vi "rsidr_core_global.vi"() -> ()   [LabVIEW 2020, in "Rohde&Schwarz RTx Oscilloscopes.lvlib"] (continued)
"Data Type"=0, "Command"="", "Access"=0, "Range Table"="", "Read Callback"="", "Write Callback"="", "Supported Models"="", "Instrument Options"="", "Flags"=0, "Help"="Current harmonics measurement total harmonic distortion results."}, {"Level"=4, "Class Only"=FALSE, "Identifier"="RSRTX_ATTR_POWER_CURRENT_HARMONICS_MEASUREMENT_TOTAL_HARMONIC_DISTORTION_CURRENT", "Descriptive Name"="Power Current Harmonics Measurement Total Harmonic Distortion Current", "Data Type"=1, "Command"="POW:HARM:MEAS:THD?", "Access"=0, "Range Table"="", "Read Callback"="", "Write Callback"="", "Supported Models"="RTM|RTA", "Instrument Options"="", "Flags"=0, "Help"="Returns the current total harmonic disortion value.\n\nAvailable Repeated Capabilities:\nNone\n\nRemote-control command(s):\nPOWer:HARMonics:MEASurement:THDistortion[:ACTual]?"}, {"Level"=4, "Class Only"=FALSE, "Identifier"="RSRTX_ATTR_POWER_CURRENT_HARMONICS_MEASUREMENT_TOTAL_HARMONIC_DISTORTION_AVERAGE", "Descriptive Name"="Power Current Harmonics Measurement Total Harmonic Distortion Average", "Data Type"=1, "Command"="POW:HARM:MEAS:THD:AVG?", "Access"=0, "Range Table"="", "Read Callback"="", "Write Callback"="", "Supported Models"="RTM|RTA", "Instrument Options"="", "Flags"=0, "Help"="Returns the average total harmonic disortion of the measured signal.\n\nAvailable Repeated Capabilities:\nNone\n\nRemote-control command(s):\nPOWer:HARMonics:MEASurement:THDistortion:AVG?"}, {"Level"=4, "Class Only"=FALSE, "Identifier"="RSRTX_ATTR_POWER_CURRENT_HARMONICS_MEASUREMENT_TOTAL_HARMONIC_DISTORTION_MAXIMUM", "Descriptive Name"="Power Current Harmonics Measurement Total Harmonic Distortion Maximum", "Data Type"=1, "Command"="POW:HARM:MEAS:THD:PPE?", "Access"=0, "Range Table"="", "Read Callback"="", "Write Callback"="", "Supported Models"="RTM|RTA", "Instrument Options"="", "Flags"=0, "Help"="Returns the maximum total harmonic disortion of the measured signal.\n\nAvailable Repeated Capabilities:\nNone\n\nRemote-control command(s):\nPOWer:HARMonics:MEASurement:THDistortion:PPEak?"}, {"Level"=4, "Class Only"=FALSE, "Identifier"="RSRTX_ATTR_POWER_CURRENT_HARMONICS_MEASUREMENT_TOTAL_HARMONIC_DISTORTION_MINIMUM", "Descriptive Name"="Power Current Harmonics Measurement Total Harmonic Distortion Minimum", "Data Type"=1, "Command"="POW:HARM:MEAS:THD:NPE?", "Access"=0, "Range Table"="", "Read Callback"="", "Write Callback"="", "Supported Models"="RTM|RTA", "Instrument Options"="", "Flags"=0, "Help"="Returns the minimum total harmonic disortion of the measured signal.\n\nAvailable Repeated Capabilities:\nNone\n\nRemote-control command(s):\nPOWer:HARMonics:MEASurement:THDistortion:NPEak?"}, {"Level"=4, "Class Only"=FALSE, "Identifier"="RSRTX_ATTR_POWER_CURRENT_HARMONICS_MEASUREMENT_TOTAL_HARMONIC_DISTORTION_STANDARD_DEVIATION", "Descriptive Name"="Power Current Harmonics Measurement Total Harmonic Distortion Standard Deviation", "Data Type"=1, "Command"="POW:HARM:MEAS:THD:STDD?", "Access"=0, "Range Table"="", "Read Callback"="", "Write Callback"="", "Supported Models"="RTM|RTA", "Instrument Options"="", "Flags"=0, "Help"="Returns the standard deviation of total harmonic disortions of the measured signal.\n\nAvailable Repeated Capabilities:\nNone\n\nRemote-control command(s):\nPOWer:HARMonics:MEASurement:THDistortion:STDDev?"}, {"Level"=3, "Class Only"=TRUE, "Identifier"="", "Descriptive Name"="Current Harmonics Export", "Data Type"=0, "Command"="", "Access"=0, "Range Table"="", "Read Callback"="", "Write Callback"="", "Supported Models"="", "Instrument Options"="", "Flags"=0, "Help"="Contains attributes for eporting power measurement."}, {"Level"=4, "Class Only"=FALSE, "Identifier"="RSRTX_ATTR_CURRENT_HARMONICS_EXPORT_NAME", "Descriptive Name"="Current Harmonics Export Name", "Data Type"=2, "Command"="EXP:POW:NAME", "Access"=2, "Range Table"="", "Read Callback"="", "Write Callback"="", "Supported Models"="RTM|RTA", "Instrument Options"="", "Flags"=0, "Help"="Defines the path and filename of the results file, available for current harmonics and spectrum power measurements. The file format is CSV. If the file already exists, it will be overwritten.\n\nAvailable Repeated Capabilities:\nNone\n\nRemote-control command(s):\nEXPort:POWer:NAME"}, {"Level"=4, "Class Only"=FALSE, "Identifier"="RSRTX_ATTR_CURRENT_HARMONICS_EXPORT_SAVE", "Descriptive Name"="Current Harmonics Export Save", "Data Type"=4, "Command"="EXP:POW:SAVE", "Access"=1, "Range Table"="", "Read Callback"="", "Write Callback"="", "Supported Models"="RTM|RTA", "Instrument Options"="", "Flags"=0, "Help"="Saves statistical results of the indicated measurement place to the file that is defined by RSRTX_ATTR_CURRENT_HARMONICS_EXPORT_NAME.\n\nAvailable Repeated Capabilities:\nNone\n\nRemote-control command(s):\nEXPort:POWer:SAVE"}, {"Level"=2, "Class Only"=TRUE, "Identifier"="", "Descriptive Name"="Inrush Current Measurement", "Data Type"=0, "Command"="", "Access"=0, "Range Table"="", "Read Callback"="", "Write Callback"="", "Supported Models"="", "Instrument Options"="", "Flags"=0, "Help"="Inrush current measurement."}, {"Level"=3, "Class Only"=FALSE, "Identifier"="RSRTX_ATTR_START_POWER_INRUSH_CURRENT_MEASUREMENT", "Descriptive Name"="Start Power Inrush Current Measurement", "Data Type"=4, "Command"="POW:INR:EXEC", "Access"=1, "Range Table"="", "Read Callback"="", "Write Callback"="", "Supported Models"="RTM|RTA", "Instrument Options"="", "Flags"=0, "Help"="Start power inrush current measurement.\n\nAvailable Repeated Capabilities:\nNone\n\nRemote-control command(s):\nPOWer:INRushcurrent:EXECute"}, {"Level"=3, "Class Only"=FALSE, "Identifier"="RSRTX_ATTR_POWER_INRUSH_CURRENT_MEASUREMENT_GATE_COUNT", "Descriptive Name"="Power Inrush Current Measurement Gate Count", "Data Type"=0, "Command"="POW:INR:GCO", "Access"=2, "Range Table"="", "Read Callback"="", "Write Callback"="", "Supported Models"="RTM|RTA", "Instrument Options"="", "Flags"=0, "Help"="Power inrush current measurement gate count.\n\nAvailable Repeated Capabilities:\nNone\n\nRemote-control command(s):\nPOWer:INRushcurrent:GCOunt"}, {"Level"=3, "Class Only"=FALSE, "Identifier"="RSRTX_ATTR_POWER_INRUSH_CURRENT_MEASUREMENT_ADD_REPORT", "Descriptive Name"="Power Inrush Current Measurement Add Report", "Data Type"=4, "Command"="POW:INR:REP:ADD", "Access"=1, "Range Table"="", "Read Callback"="", "Write Callback"="", "Supported Models"="RTM|RTA", "Instrument Options"="", "Flags"=1, "Help"="Adds the result to the report list.\n\nAvailable Repeated Capabilities:\nNone\n\nRemote-control command(s):\nPOWer:INRushcurrent:REPort:ADD"}, {"Level"=3, "Class Only"=TRUE, "Identifier"="", "Descriptive Name"="Gate", "Data Type"=0, "Command"="", "Access"=0, "Range Table"="", "Read Callback"="", "Write Callback"="", "Supported Models"="", "Instrument Options"="", "Flags"=0, "Help"="Attributes with gate repeated capability."}, {"Level"=4, "Class Only"=FALSE, "Identifier"="RSRTX_ATTR_POWER_INRUSH_CURRENT_MEASUREMENT_GATE_START", "Descriptive Name"="Power Inrush Current Measurement Gate Start", "Data Type"=1, "Command"="POW:INR:GATE{Gate}:STAR", "Access"=2, "Range Table"="", "Read Callback"="", "Write Callback"="", "Supported Models"="RTM|RTA", "Instrument Options"="", "Flags"=0, "Help"="Start of the gate.\n\nAvailable Repeated Capabilities:\nGate: Gate1, Gate2, Gate3\r\n\nRemote-control command(s):\nPOWer:INRushcurrent:GATE<n>:STARt"}, {"Level"=4, "Class Only"=FALSE, "Identifier"="RSRTX_ATTR_POWER_INRUSH_CURRENT_MEASUREMENT_GATE_STOP", "Descriptive Name"="Power Inrush Current Measurement Gate Stop", "Data Type"=1, "Command"="POW:INR:GATE{Gate}:STOP", "Access"=2, "Range Table"="", "Read Callback"="", "Write Callback"="", "Supported Models"="RTM|RTA", "Instrument Options"="", "Flags"=0, "Help"="Stop of the gate.\n\nAvailable Repeated Capabilities:\nGate: Gate1, Gate2, Gate3\r\n\nRemote-control command(s):\nPOWer:INRushcurrent:GATE<n>:STOP"}, {"Level"=3, "Class Only"=TRUE, "Identifier"="", "Descriptive Name"="Results", "Data Type"=0, "Command"="", "Access"=0, "Range Table"="", "Read Callback"="", "Write Callback"="", "Supported Models"="", "Instrument Options"="", "Flags"=0, "Help"="Results of the inrush current measurement."}, {"Level"=4, "Class Only"=FALSE, "Identifier"="RSRTX_ATTR_POWER_INRUSH_CURRENT_MEASUREMENT_AREA_RESULT", "Descriptive Name"="Power Inrush Current Measurement Area Result", "Data Type"=1, "Command"="POW:INR:RES{Gate}:AREA?", "Access"=0, "Range Table"="", "Read Callback"="", "Write Callback"="", "Supported Models"="RTM|RTA", "Instrument Options"="", "Flags"=0, "Help"="Area result of the measurement.\n\nAvailable Repeated Capabilities:\nGate: Gate1, Gate2, Gate3\r\n\nRemote-control command(s):\nPOWer:INRushcurrent:RESult<n>:AREA?"}, {"Level"=4, "Class Only"=FALSE, "Identifier"="RSRTX_ATTR_POWER_INRUSH_CURRENT_MEASUREMENT_MAXIMUM_RESULT", "Descriptive Name"="Power Inrush Current Measurement Maximum Result", "Data Type"=1, "Command"="POW:INR:RES{Gate}:MAXCurrent?", "Access"=0, "Range Table"="", "Read Callback"="", "Write Callback"="", "Supported Models"="RTM|RTA", "Instrument Options"="", "Flags"=0, "Help"="Maximum result of the measurement.\n\nAvailable Repeated Capabilities:\nGate: Gate1, Gate2, Gate3\r\n\nRemote-control command(s):\nPOWer:INRushcurrent:RESult<n>:MAXCurrent?"}, {"Level"=2, "Class Only"=TRUE, "Identifier"="", "Descriptive Name"="Ripple Measurement", "Data Type"=0, "Command"="", "Access"=0, "Range Table"="", "Read Callback"="", "Write Callback"="", "Supported Models"="", "Instrument Options"="", "Flags"=0, "Help"="Ripple mesurement."}, {"Level"=3, "Class Only"=FALSE, "Identifier"="RSRTX_ATTR_START_POWER_RIPPLE_MEASUREMENT", "Descriptive Name"="Start Power Ripple Measurement", "Data Type"=4, "Command"="POW:RIPP:EXEC", "Access"=1, "Range Table"="", "Read Callback"="", "Write Callback"="", "Supported Models"="RTM|RTA", "Instrument Options"="", "Flags"=0, "Help"="Start power ripple measurement.\n\nAvailable Repeated Capabilities:\nNone\n\nRemote-control command(s):\nPOWer:RIPPle:EXECute"}, {"Level"=3, "Class Only"=FALSE, "Identifier"="RSRTX_ATTR_POWER_RIPPLE_MEASUREMENT_ADD_REPORT", "Descriptive Name"="Power Ripple Measurement Add Report", "Data Type"=4, "Command"="POW:RIPP:REP:ADD", "Access"=1, "Range Table"="", "Read Callback"="", "Write Callback"="", "Supported Models"="RTM|RTA", "Instrument Options"="", "Flags"=1, "Help"="Adds the result to the report list.\n\nAvailable Repeated Capabilities:\nNone\n\nRemote-control command(s):\nPOWer:RIPPle:REPort:ADD"}, {"Level"=3, "Class Only"=TRUE, "Identifier"="", "Descriptive Name"="Results", "Data Type"=0, "Command"="", "Access"=0, "Range Table"="", "Read Callback"="", "Write Callback"="", "Supported Models"="", "Instrument Options"="", "Flags"=0, "Help"="Results of the ripple analysis."}, {"Level"=2, "Class Only"=TRUE, "Identifier"="", "Descriptive Name"="Spectrum Measurement", "Data Type"=0, "Command"="", "Access"=0, "Range Table"="", "Read Callback"="", "Write Callback"="", "Supported Models"="", "Instrument Options"="", "Flags"=0, "Help"="Power spectrum measurement."}, {"Level"=3, "Class Only"=FALSE, "Identifier"="RSRTX_ATTR_START_POWER_SPECTRUM_MEASUREMENT", "Descriptive Name"="Start Power Spectrum Measurement", "Data Type"=4, "Command"="POW:SPEC:EXEC", "Access"=1, "Range Table"="", "Read Callback"="", "Write Callback"="", "Supported Models"="RTM|RTA", "Instrument Options"="", "Flags"=1, "Help"="Starts the spectrum measurement.\n\nAvailable Repeated Capabilities:\nNone\n\nRemote-control command(s):\nPOWer:SPECtrum:EXECute"}, {"Level"=3, "Class Only"=FALSE, "Identifier"="RSRTX_ATTR_POWER_SPECTRUM_MEASUREMENT_FREQUENCY", "Descriptive Name"="Power Spectrum Measurement Frequency", "Data Type"=1, "Command"="POW:SPEC:FREQ", "Access"=2, "Range Table"="", "Read Callback"="", "Write Callback"="", "Supported Models"="RTM|RTA", "Instrument Options"="", "Flags"=0, "Help"="Sets the SMPS switching frequency.\n\nAvailable Repeated Capabilities:\nNone\n\nRemote-control command(s):\nPOWer:SPECtrum:FREQuency"}, {"Level"=3, "Class Only"=FALSE, "Identifier"="RSRTX_ATTR_POWER_SPECTRUM_MEASUREMENT_ADD_REPORT", "Descriptive Name"="Power Spectrum Measurement Add Report", "Data Type"=4, "Command"="POW:SPEC:REP:ADD", "Access"=1, "Range Table"="", "Read Callback"="", "Write Callback"="", "Supported Models"="RTM|RTA", "Instrument Options"="", "Flags"=1, "Help"="Adds the result to the report list.\n\nAvailable Repeated Capabilities:\nNone\n\nRemote-control command(s):\nPOWer:SPECtrum:REPort:ADD"}, {"Level"=3, "Class Only"=TRUE, "Identifier"="", "Descriptive Name"="Results", "Data Type"=0, "Command"="", "Access"=0, "Range Table"="", "Read Callback"="", "Write Callback"="", "Supported Models"="", "Instrument Options"="", "Flags"=0, "Help"="Power Spectrum Measurement Results."}, {"Level"=4, "Class Only"=FALSE, "Identifier"="RSRTX_ATTR_RESET_POWER_SPECTRUM_MEASUREMENT_RESULTS", "Descriptive Name"="Reset Power Spectrum Measurement Results", "Data Type"=4, "Command"="POW:SPEC:RES{ResultNumber}:RES", "Access"=1, "Range Table"="", "Read Callback"="", "Write Callback"="", "Supported Models"="RTM|RTA", "Instrument Options"="", "Flags"=0, "Help"="Resets the results.\n\nAvailable Repeated Capabilities:\nResultNumber: Res1, Res2, Res3, Res4, Res5, Res6, Res7, Res8, Res9, Res10, Res11, Res12, Res13, Res14, Res15, Res16, Res17, Res18, Res19, Res20, Res21, Res22, Res23, Res24, Res25, Res26, Res27, Res28, Res29, Res30, Res31, Res32, Res33, Res34, Res35, Res36, Res37, Res38, Res39, Res40\r\n\nRemote-control command(s):\nPOWer:SPECtrum:RESult<n>:RESet"}, {"Level"=2, "Class Only"=TRUE, "Identifier"="", "Descriptive Name"="Slew Rate Measurement", "Data Type"=0, "Command"="", "Access"=0, "Range Table"="", "Read Callback"="", "Write Callback"="", "Supported Models"="", "Instrument Options"="", "Flags"=0, "Help"="Slew rate measurement."}, {"Level"=3, "Class Only"=FALSE, "Identifier"="RSRTX_ATTR_START_POWER_SLEW_RATE_MEASUREMENT", "Descriptive Name"="Start Power Slew Rate Measurement", "Data Type"=4, "Command"="POW:SLEW:EXEC", "Access"=1, "Range Table"="", "Read Callback"="", "Write Callback"="", "Supported Models"="RTM|RTA", "Instrument Options"="", "Flags"=0, "Help"="Starts the slew rate measurement.\n\nAvailable Repeated Capabilities:\nNone\n\nRemote-control command(s):\nPOWer:SLEWrate:EXECute"}, {"Level"=3, "Class Only"=FALSE, "Identifier"="RSRTX_ATTR_POWER_SLEW_RATE_MEASUREMENT_DELTA_SAMPLE", "Descriptive Name"="Power Slew Rate Measurement Delta Sample", "Data Type"=1, "Command"="POW:SLEW:DSAM", "Access"=2, "Range Table"="", "Read Callback"="", "Write Callback"="", "Supported Models"="RTM|RTA", "Instrument Options"="", "Flags"=0, "Help"="Configures the length of the delta sample\n\nAvailable Repeated Capabilities:\nNone\n\nRemote-control command(s):\nPOWer:SLEWrate:DSAMple"}, {"Level"=3, "Class Only"=FALSE, "Identifier"="RSRTX_ATTR_POWER_SLEW_RATE_MEASUREMENT_DELTA_TIME", "Descriptive Name"="Power Slew Rate Measurement Delta Time", "Data Type"=1, "Command"="POW:SLEW:DTIM", "Access"=2, "Range Table"="", "Read Callback"="", "Write Callback"="", "Supported Models"="RTM|RTA", "Instrument Options"="", "Flags"=0, "Help"="Configures the delta time.\n\nAvailable Repeated Capabilities:\nNone\n\nRemote-control command(s):\nPOWer:SLEWrate:DTIMe"}, {"Level"=3, "Class Only"=FALSE, "Identifier"="RSRTX_ATTR_POWER_SLEW_RATE_MEASUREMENT_ADD_REPORT", "Descriptive Name"="Power Slew Rate Measurement Add Report", "Data Type"=4, "Command"="POW:SLEW:REP:ADD", "Access"=1, "Range Table"="", "Read Callback"="", "Write Callback"="", "Supported Models"="RTM|RTA", "Instrument Options"="", "Flags"=1, "Help"="Adds the result to the report list.\n\nAvailable Repeated Capabilities:\nNone\n\nRemote-control command(s):\nPOWer:SLEWrate:REPort:ADD"}, {"Level"=3, "Class Only"=TRUE, "Identifier"="", "Descriptive Name"="Results", "Data Type"=0, "Command"="", "Access"=0, "Range Table"="", "Read Callback"="", "Write Callback"="", "Supported Models"="", "Instrument Options"="", "Flags"=0, "Help"="Slew rate measurement results."}, {"Level"=2, "Class Only"=TRUE, "Identifier"="", "Descriptive Name"="Modulation Measurement", "Data Type"=0, "Command"="", "Access"=0, "Range Table"="", "Read Callback"="", "Write Callback"="", "Supported Models"="", "Instrument Options"="", "Flags"=0, "Help"="Power modulation measurement."}, {"Level"=3, "Class Only"=FALSE, "Identifier"="RSRTX_ATTR_START_POWER_MODULATION_MEASUREMENT", "Descriptive Name"="Start Power Modulation Measurement", "Data Type"=4, "Command"="POW:MOD:EXEC", "Access"=1, "Range Table"="", "Read Callback"="", "Write Callback"="", "Supported Models"="RTM|RTA", "Instrument Options"="", "Flags"=0, "Help"="Starts the measurement.\n\nAvailable Repeated Capabilities:\nNone\n\nRemote-control command(s):\nPOWer:MODulation:EXECute"}, {"Level"=3, "Class Only"=FALSE, "Identifier"="RSRTX_ATTR_POWER_MODULATION_MEASUREMENT_TYPE", "Descriptive Name"="Power Modulation Measurement Type", "Data Type"=0, "Command"="POW:MOD:TYPE", "Access"=2, "Range Table"="rsrtx_rngModulationType", "Read Callback"="", "Write Callback"="", "Supported Models"="RTM|RTA", "Instrument Options"="", "Flags"=0, "Help"="Selects modulation type.\n\nAvailable Repeated Capabilities:\nNone\n\nRemote-control command(s):\nPOWer:MODulation:TYPE"}, {"Level"=3, "Class Only"=FALSE, "Identifier"="RSRTX_ATTR_POWER_MODULATION_MEASUREMENT_ADD_REPORT", "Descriptive Name"="Power Modulation Measurement Add Report", "Data Type"=4, "Command"="POW:MOD:REP:ADD", "Access"=1, "Range Table"="", "Read Callback"="", "Write Callback"="", "Supported Models"="RTM|RTA", "Instrument Options"="", "Flags"=1, "Help"="Adds the result to the report list.\n\nAvailable Repeated Capabilities:\nNone\n\nRemote-control command(s):\nPOWer:MODulation:REPort:ADD"}, {"Level"=3, "Class Only"=FALSE, "Identifier"="RSRTX_ATTR_POWER_MODULATION_THRESHOLD_UPPER", "Descriptive Name"="Power Modulation Threshold Upper", "Data Type"=1, "Command"="POW:MOD:THR", "Access"=2, "Range Table"="", "Read Callback"="", "Write Callback"="", "Supported Models"="", "Instrument Options"="", "Flags"=0, "Help"="Sets the threshold for unipolar sources, or the upper level for bipolar sources. The signal is measured at the crossing points of the signal with the threshold.\n\nAvailable Repeated Capabilities:\nNone\n\nRemote-control command(s):\nPOWer:MODulation:THReshold[:UPPer]"}, {"Level"=3, "Class Only"=FALSE, "Identifier"="RSRTX_ATTR_POWER_MODULATION_THRESHOLD_LOWER", "Descriptive Name"="Power Modulation Threshold Lower", "Data Type"=1, "Command"="POW:MOD:THR:LOW", "Access"=2, "Range Table"="", "Read Callback"="", "Write Callback"="", "Supported Models"="", "Instrument Options"="", "Flags"=0, "Help"="Sets the lower level for bipolar sources, which determines the crossing points on negative pulses.\n\nAvailable Repeated Capabilities:\nNone\n\nRemote-control command(s):\nPOWer:MODulation:THReshold:LOWer"}, {"Level"=3, "Class Only"=FALSE, "Identifier"="RSRTX_ATTR_POWER_MODULATION_THRESHOLD_HYSTERESIS", "Descriptive Name"="Power Modulation Threshold Hysteresis", "Data Type"=1, "Command"="POW:MOD:THR:HYST", "Access"=2, "Range Table"="", "Read Callback"="", "Write Callback"="", "Supported Models"="", "Instrument Options"="", "Flags"=0, "Help"="Sets the hysteresis for correct edge detection.\n\nAvailable Repeated Capabilities:\nNone\n\nRemote-control command(s):\nPOWer:MODulation:THReshold:HYSTeresis"}, {"Level"=3, "Class Only"=TRUE, "Identifier"="", "Descriptive Name"="Results", "Data Type"=0, "Command"="", "Access"=0, "Range Table"="", "Read Callback"="", "Write Callback"="", "Supported Models"="", "Instrument Options"="", "Flags"=0, "Help"="Results of the modulation measurement."}, {"Level"=2, "Class Only"=TRUE, "Identifier"="", "Descriptive Name"="Dynamic On Resistance Measurement", "Data Type"=0, "Command"="", "Access"=0, "Range Table"="", "Read Callback"="", "Write Callback"="", "Supported Models"="", "Instrument Options"="", "Flags"=0, "Help"="Dynamic On Resistance Measurement."}, {"Level"=3, "Class Only"=FALSE, "Identifier"="RSRTX_ATTR_START_POWER_DYNAMIC_ON_RESISTANCE_MEASUREMENT", "Descriptive Name"="Start Power Dynamic On Resistance Measurement", "Data Type"=4, "Command"="POW:DONR:EXEC", "Access"=1, "Range Table"="", "Read Callback"="", "Write Callback"="", "Supported Models"="RTM|RTA", "Instrument Options"="", "Flags"=0, "Help"="Starts the measurement.\n\nAvailable Repeated Capabilities:\nNone\n\nRemote-control command(s):\nPOWer:DONResistance:EXECute"}, {"Level"=3, "Class Only"=FALSE, "Identifier"="RSRTX_ATTR_POWER_DYNAMIC_ON_RESISTANCE_MEASUREMENT_ADD_REPORT", "Descriptive Name"="Power Dynamic On Resistance Measurement Add Report", "Data Type"=4, "Command"="POW:DONR:REP:ADD", "Access"=1, "Range Table"="", "Read Callback"="", "Write Callback"="", "Supported Models"="RTM|RTA", "Instrument Options"="", "Flags"=1, "Help"="Adds the result to the report list.\n\nAvailable Repeated Capabilities:\nNone\n\nRemote-control command(s):\nPOWer:DONResistance:REPort:ADD"}, {"Level"=3, "Class Only"=TRUE, "Identifier"="", "Descriptive Name"="Gate", "Data Type"=0, "Command"="", "Access"=0, "Range Table"="", "Read Callback"="", "Write Callback"="", "Supported Models"="", "Instrument Options"="", "Flags"=0, "Help"="Attributes with gate repeated capability."}, {"Level"=4, "Class Only"=FALSE, "Identifier"="RSRTX_ATTR_POWER_DYNAMIC_ON_RESISTANCE_MEASUREMENT_GATE_START", "Descriptive Name"="Power Dynamic On Resistance Measurement Gate Start", "Data Type"=1, "Command"="POW:DONR:GATE{Gate}:START", "Access"=2, "Range Table"="", "Read Callback"="", "Write Callback"="", "Supported Models"="RTM|RTA", "Instrument Options"="", "Flags"=0, "Help"="Start of the gate.\n\nAvailable Repeated Capabilities:\nGate: Gate1, Gate2, Gate3\r\n\nRemote-control command(s):\nPOWer:DONResistance:GATE<n>:START"}, {"Level"=4, "Class Only"=FALSE, "Identifier"="RSRTX_ATTR_POWER_DYNAMIC_ON_RESISTANCE_MEASUREMENT_GATE_STOP", "Descriptive Name"="Power Dynamic On Resistance Measurement Gate Stop", "Data Type"=1, "Command"="POW:DONR:GATE{Gate}:STOP", "Access"=2, "Range Table"="", "Read Callback"="", "Write Callback"="", "Supported Models"="RTM|RTA", "Instrument Options"="", "Flags"=0, "Help"="Stop of the gate.\n\nAvailable Repeated Capabilities:\nGate: Gate1, Gate2, Gate3\r\n\nRemote-control command(s):\nPOWer:DONResistance:GATE<n>STOP"}, {"Level"=3, "Class Only"=TRUE, "Identifier"="", "Descriptive Name"="Results", "Data Type"=0, "Command"="", "Access"=0, "Range Table"="", "Read Callback"="", "Write Callback"="", "Supported Models"="", "Instrument Options"="", "Flags"=0, "Help"="Provides the results of dynamic on resistance measurement."}, {"Level"=4, "Class Only"=FALSE, "Identifier"="RSRTX_ATTR_POWER_DYNAMIC_ON_RESISTANCE_MEASUREMENT_RESULT", "Descriptive Name"="Power Dynamic On Resistance Measurement Result", "Data Type"=1, "Command"="POW:DONR:RES:DONR?", "Access"=0, "Range Table"="", "Read Callback"="", "Write Callback"="", "Supported Models"="RTM|RTA", "Instrument Options"="", "Flags"=0, "Help"="Returns the result of the measurement\n\nAvailable Repeated Capabilities:\nNone\n\nRemote-control command(s):\nPOWer:DONResistance:RESult:DONResistance?"}, {"Level"=2, "Class Only"=TRUE, "Identifier"="", "Descriptive Name"="Efficiency Measurement", "Data Type"=0, "Command"="", "Access"=0, "Range Table"="", "Read Callback"="", "Write Callback"="", "Supported Models"="", "Instrument Options"="", "Flags"=0, "Help"="Power efficiency measurement."}, {"Level"=3, "Class Only"=FALSE, "Identifier"="RSRTX_ATTR_START_POWER_EFFICIENCY_MEASUREMENT", "Descriptive Name"="Start Power Efficiency Measurement", "Data Type"=4, "Command"="POW:EFF:EXEC", "Access"=1, "Range Table"="", "Read Callback"="", "Write Callback"="", "Supported Models"="RTM|RTA", "Instrument Options"="", "Flags"=0, "Help"="Starts the measurement.\n\nAvailable Repeated Capabilities:\nNone\n\nRemote-control command(s):\nPOWer:EFFiciency:EXECute"}, {"Level"=3, "Class Only"=FALSE, "Identifier"="RSRTX_ATTR_POWER_EFFICIENCY_MEASUREMENT_ADD_REPORT", "Descriptive Name"="Power Efficiency Measurement Add Report", "Data Type"=4, "Command"="POW:EFF:REP:ADD", "Access"=1, "Range Table"="", "Read Callback"="", "Write Callback"="", "Supported Models"="RTM|RTA", "Instrument Options"="", "Flags"=1, "Help"="Adds the result to the report list.\n\nAvailable Repeated Capabilities:\nNone\n\nRemote-control command(s):\nPOWer:EFFiciency:REPort:ADD"}, {"Level"=3, "Class Only"=TRUE, "Identifier"="", "Descriptive Name"="Results", "Data Type"=0, "Command"="", "Access"=0, "Range Table"="", "Read Callback"="", "Write Callback"="", "Supported Models"="", "Instrument Options"="", "Flags"=0, "Help"="Results of the measurement."}, {"Level"=2, "Class Only"=TRUE, "Identifier"="", "Descriptive Name"="Switchingloss Measurement", "Data Type"=0, "Command"="", "Access"=0, "Range Table"="", "Read Callback"="", "Write Callback"="", "Supported Models"="", "Instrument Options"="", "Flags"=0, "Help"="Switchingloss measurement"}, {"Level"=3, "Class Only"=FALSE, "Identifier"="RSRTX_ATTR_START_POWER_SWITCHINGLOSS_MEASUREMENT", "Descriptive Name"="Start Power Switchingloss Measurement", "Data Type"=4, "Command"="POW:SWIT:EXEC", "Access"=1, "Range Table"="", "Read Callback"="", "Write Callback"="", "Supported Models"="RTM|RTA", "Instrument Options"="", "Flags"=0, "Help"="Starts the measurement.\n\nAvailable Repeated Capabilities:\nNone\n\nRemote-control command(s):\nPOWer:SWITching:EXECute"}, {"Level"=3, "Class Only"=FALSE, "Identifier"="RSRTX_ATTR_POWER_SWITCHINGLOSS_MEASUREMENT_TYPE", "Descriptive Name"="Power Switchingloss Measurement Type", "Data Type"=0, "Command"="POW:SWIT:TYPE", "Access"=2, "Range Table"="rsrtx_rngSwitchinglossType", "Read Callback"="", "Write Callback"="", "Supported Models"="RTM|RTA", "Instrument Options"="", "Flags"=0, "Help"="Configures switchingloss measurement type.\n\nAvailable Repeated Capabilities:\nNone\n\nRemote-control command(s):\nPOWer:SWITching:TYPE"}, {"Level"=3, "Class Only"=FALSE, "Identifier"="RSRTX_ATTR_POWER_SWITCHINGLOSS_MEASUREMENT_ADD_REPORT", "Descriptive Name"="Power Switchingloss Measurement Add Report", "Data Type"=4, "Command"="POW:SWIT:REP:ADD", "Access"=1, "Range Table"="", "Read Callback"="", "Write Callback"="", "Supported Models"="RTM|RTA", "Instrument Options"="", "Flags"=1, "Help"="Adds the result to the report list.\n\nAvailable Repeated Capabilities:\nNone\n\nRemote-control command(s):\nPOWer:SWITching:REPort:ADD"}, {"Level"=3, "Class Only"=TRUE, "Identifier"="", "Descriptive Name"="Gate", "Data Type"=0, "Command"="", "Access"=0, "Range Table"="", "Read Callback"="", "Write Callback"="", "Supported Models"="", "Instrument Options"="", "Flags"=0, "Help"="Configures gate."}, {"Level"=4, "Class Only"=FALSE, "Identifier"="RSRTX_ATTR_SET_POWER_SWITSCHINGLOSS_MEASUREMENT_GATE_TO_WAVEFORM", "Descriptive Name"="Set Power Switschingloss Measurement Gate To Waveform", "Data Type"=4, "Command"="POW:SWIT:SWAV", "Access"=1, "Range Table"="", "Read Callback"="", "Write Callback"="", "Supported Models"="RTM|RTA", "Instrument Options"="", "Flags"=0, "Help"="Sets gate to waveform.\n\nAvailable Repeated Capabilities:\nNone\n\nRemote-control command(s):\nPOWer:SWITching:GATE:SWAVe"}, {"Level"=4, "Class Only"=FALSE, "Identifier"="RSRTX_ATTR_POWER_SWITCHINGLOSS_MEASUREMENT_GATE_CONDUCTION_START", "Descriptive Name"="Power Switchingloss Measurement Gate Conduction Start", "Data Type"=1, "Command"="POW:SWIT:GATE:COND:STAR", "Access"=2, "Range Table"="", "Read Callback"="", "Write Callback"="", "Supported Models"="RTM|RTA", "Instrument Options"="", "Flags"=0, "Help"="Start of the gate.\n\nAvailable Repeated Capabilities:\nNone\n\nRemote-control command(s):\nPOWer:SWITching:GATE:CONDuction:STARt"}, {"Level"=4, "Class Only"=FALSE, "Identifier"="RSRTX_ATTR_POWER_SWITCHINGLOSS_MEASUREMENT_GATE_CONDUCTION_STOP", "Descriptive Name"="Power Switchingloss Measurement Gate Conduction Stop", "Data Type"=1, "Command"="POW:SWIT:GATE:COND:STOP", "Access"=2, "Range Table"="", "Read Callback"="", "Write Callback"="", "Supported Models"="RTM|RTA", "Instrument Options"="", "Flags"=0, "Help"="Stop of the gate.\n\nAvailable Repeated Capabilities:\nNone\n\nRemote-control command(s):\nPOWer:SWITching:GATE:CONDuction:STOP"}, {"Level"=4, "Class Only"=FALSE, "Identifier"="RSRTX_ATTR_POWER_SWITCHINGLOSS_MEASUREMENT_GATE_NO_CONDUCTION_START", "Descriptive Name"="Power Switchingloss Measurement Gate No Conduction Start", "Data Type"=1, "Command"="POW:SWIT:GATE:NCON:STAR", "Access"=2, "Range Table"="", "Read Callback"="", "Write Callback"="", "Supported Models"="RTM|RTA", "Instrument Options"="", "Flags"=0, "Help"="Start of the gate.\n\nAvailable Repeated Capabilities:\nNone\n\nRemote-control command(s):\nPOWer:SWITching:GATE:NCONduction:STARt"}, {"Level"=4, "Class Only"=FALSE, "Identifier"="RSRTX_ATTR_POWER_SWITCHINGLOSS_MEASUREMENT_GATE_NO_CONDUCTION_STOP", "Descriptive Name"="Power Switchingloss Measurement Gate No Conduction Stop", "Data Type"=1, "Command"="POW:SWIT:GATE:NCON:STOP", "Access"=2, "Range Table"="", "Read Callback"="", "Write Callback"="", "Supported Models"="RTM|RTA", "Instrument Options"="", "Flags"=0, "Help"="Stop of the gate.\n\nAvailable Repeated Capabilities:\nNone\n\nRemote-control command(s):\nPOWer:SWITching:GATE:NCONduction:STOP"}, {"Level"=4, "Class Only"=FALSE, "Identifier"="RSRTX_ATTR_POWER_SWITCHINGLOSS_MEASUREMENT_GATE_TURN_ON_START", "Descriptive Name"="Power Switchingloss Measurement Gate Turn On Start", "Data Type"=1, "Command"="POW:SWIT:GATE:TON:STAR", "Access"=2, "Range Table"="", "Read Callback"="", "Write Callback"="", "Supported Models"="RTM|RTA", "Instrument Options"="", "Flags"=0, "Help"="Start of the gate.\n\nAvailable Repeated Capabilities:\nNone\n\nRemote-control command(s):\nPOWer:SWITching:GATE:TON:STARt"}, {"Level"=4, "Class Only"=FALSE, "Identifier"="RSRTX_ATTR_POWER_SWITCHINGLOSS_MEASUREMENT_GATE_TURN_ON_STOP", "Descriptive Name"="Power Switchingloss Measurement Gate Turn On Stop", "Data Type"=1, "Command"="POW:SWIT:GATE:TON:STOP", "Access"=2, "Range Table"="", "Read Callback"="", "Write Callback"="", "Supported Models"="RTM|RTA", "Instrument Options"="", "Flags"=0, "Help"="Stop of the gate.\n\nAvailable Repeated Capabilities:\nNone\n\nRemote-control command(s):\nPOWer:SWITching:GATE:TON:STOP"}, {"Level"=4, "Class Only"=FALSE, "Identifier"="RSRTX_ATTR_POWER_SWITCHINGLOSS_MEASUREMENT_GATE_TURN_OFF_START", "Descriptive Name"="Power Switchingloss Measurement Gate Turn Off Start", "Data Type"=1, "Command"="POW:SWIT:GATE:TOFF:STAR", "Access"=2, "Range Table"="", "Read Callback"="", "Write Callback"="", "Supported Models"="RTM|RTA", "Instrument Options"="", "Flags"=0, "Help"="Start of the gate.\n\nAvailable Repeated Capabilities:\nNone\n\nRemote-control command(s):\nPOWer:SWITching:GATE:TOFF:STARt"}, {"Level"=4, "Class Only"=FALSE, "Identifier"="RSRTX_ATTR_POWER_SWITCHINGLOSS_MEASUREMENT_GATE_TURN_OFF_STOP", "Descriptive Name"="Power Switchingloss Measurement Gate Turn Off Stop", "Data Type"=1, "Command"="POW:SWIT:GATE:TOFF:STOP", "Access"=2, "Range Table"="", "Read Callback"="", "Write Callback"="", "Supported Models"="RTM|RTA", "Instrument Options"="", "Flags"=0, "Help"="Stop of the gate.\n\nAvailable Repeated Capabilities:\nNone\n\nRemote-control command(s):\nPOWer:SWITching:GATE:TOFF:STOP"}, {"Level"=3, "Class Only"=TRUE, "Identifier"="", "Descriptive Name"="Results", "Data Type"=0, "Command"="", "Access"=0, "Range Table"="", "Read Callback"="", "Write Callback"="", "Supported Models"="", "Instrument Options"="", "Flags"=0, "Help"="Results of the measurement."}, {"Level"=4, "Class Only"=FALSE, "Identifier"="RSRTX_ATTR_POWER_SWITCHINGLOSS_MEASUREMENT_CONDUCTION_ENERGY_RESULT", "Descriptive Name"="Power Switchingloss Measurement Conduction Energy Result", "Data Type"=1, "Command"="POW:SWIT:RES:COND:ENER?", "Access"=0, "Range Table"="", "Read Callback"="", "Write Callback"="", "Supported Models"="RTM|RTA", "Instrument Options"="", "Flags"=0, "Help"="Result of the measurement\n\nAvailable Repeated Capabilities:\nNone\n\nRemote-control command(s):\nPOWer:SWITching:RESult:CONDuction:ENERgy?"}, {"Level"=4, "Class Only"=FALSE, "Identifier"="RSRTX_ATTR_POWER_SWITCHINGLOSS_MEASUREMENT_CONDUCTION_POWER_RESULT", "Descriptive Name"="Power Switchingloss Measurement Conduction Power Result", "Data Type"=1, "Command"="POW:SWIT:RES:COND:POW?", "Access"=0, "Range Table"="", "Read Callback"="", "Write Callback"="", "Supported Models"="RTM|RTA", "Instrument Options"="", "Flags"=0, "Help"="Result of the measurement\n\nAvailable Repeated Capabilities:\nNone\n\nRemote-control command(s):\nPOWer:SWITching:RESult:CONDuction:POWer?"}, {"Level"=4, "Class Only"=FALSE, "Identifier"="RSRTX_ATTR_POWER_SWITCHINGLOSS_MEASUREMENT_NO_CONDUCTION_ENERGY_RESULT", "Descriptive Name"="Power Switchingloss Measurement No Conduction Energy Result", "Data Type"=1, "Command"="POW:SWIT:RES:NCON:ENER?", "Access"=0, "Range Table"="", "Read Callback"="", "Write Callback"="", "Supported Models"="RTM|RTA", "Instrument Options"="", "Flags"=0, "Help"="Result of the measurement\n\nAvailable Repeated Capabilities:\nNone\n\nRemote-control command(s):\nPOWer:SWITching:RESult:NCONduction:ENERgy?"}, {"Level"=4, "Class Only"=FALSE, "Identifier"="RSRTX_ATTR_POWER_SWITCHINGLOSS_MEASUREMENT_NO_CONDUCTION_POWER_RESULT", "Descriptive Name"="Power Switchingloss Measurement No Conduction Power Result", "Data Type"=1, "Command"="POW:SWIT:RES:NCON:POW?", "Access"=0, "Range Table"="", "Read Callback"="", "Write Callback"="", "Supported Models"="RTM|RTA", "Instrument Options"="", "Flags"=0, "Help"="Result of the measurement\n\nAvailable Repeated Capabilities:\nNone\n\nRemote-control command(s):\nPOWer:SWITching:RESult:NCONduction:POWer?"}, {"Level"=4, "Class Only"=FALSE, "Identifier"="RSRTX_ATTR_POWER_SWITCHINGLOSS_MEASUREMENT_TURN_ON_ENERGY_RESULT", "Descriptive Name"="Power Switchingloss Measurement Turn On Energy Result", "Data Type"=1, "Command"="POW:SWIT:RES:TON:ENER?", "Access"=0, "Range Table"="", "Read Callback"="", "Write Callback"="", "Supported Models"="RTM|RTA", "Instrument Options"="", "Flags"=0, "Help"="Result of the measurement\n\nAvailable Repeated Capabilities:\nNone\n\nRemote-control command(s):\nPOWer:SWITching:RESult:TON:ENERgy?"}, {"Level"=4, "Class Only"=FALSE, "Identifier"="RSRTX_ATTR_POWER_SWITCHINGLOSS_MEASUREMENT_TURN_ON_POWER_RESULT", "Descriptive Name"="Power Switchingloss Measurement Turn On Power Result", "Data Type"=1, "Command"="POW:SWIT:RES:TON:POW?", "Access"=0, "Range Table"="", "Read Callback"="", "Write Callback"="", "Supported Models"="RTM|RTA", "Instrument Options"="", "Flags"=0, "Help"="Result of the measurement\n\nAvailable Repeated Capabilities:\nNone\n\nRemote-control command(s):\nPOWer:SWITching:RESult:TON:POWer?"}, {"Level"=4, "Class Only"=FALSE, "Identifier"="RSRTX_ATTR_POWER_SWITCHINGLOSS_MEASUREMENT_TURN_OFF_ENERGY_RESULT", "Descriptive Name"="Power Switchingloss Measurement Turn Off Energy Result", "Data Type"=1, "Command"="POW:SWIT:RES:TOFF:ENER?", "Access"=0, "Range Table"="", "Read Callback"="", "Write Callback"="", "Supported Models"="RTM|RTA", "Instrument Options"="", "Flags"=0, "Help"="Result of the measurement\n\nAvailable Repeated Capabilities:\nNone\n\nRemote-control command(s):\nPOWer:SWITching:RESult:TOFF:ENERgy?"}, {"Level"=4, "Class Only"=FALSE, "Identifier"="RSRTX_ATTR_POWER_SWITCHINGLOSS_MEASUREMENT_TURN_OFF_POWER_RESULT", "Descriptive Name"="Power Switchingloss Measurement Turn Off Power Result", "Data Type"=1, "Command"="POW:SWIT:RES:TOFF:POW?", "Access"=0, "Range Table"="", "Read Callback"="", "Write Callback"="", "Supported Models"="RTM|RTA", "Instrument Options"="", "Flags"=0, "Help"="Result of the measurement\n\nAvailable Repeated Capabilities:\nNone\n\nRemote-control command(s):\nPOWer:SWITching:RESult:TOFF:POWer?"}, {"Level"=4, "Class Only"=FALSE, "Identifier"="RSRTX_ATTR_POWER_SWITCHINGLOSS_MEASUREMENT_TOTAL_ENERGY_RESULT", "Descriptive Name"="Power Switchingloss Measurement Total Energy Result", "Data Type"=1, "Command"="POW:SWIT:RES:TOT:ENER?", "Access"=0, "Range Table"="", "Read Callback"="", "Write Callback"="", "Supported Models"="RTM|RTA", "Instrument Options"="", "Flags"=0, "Help"="Result of the measurement\n\nAvailable Repeated Capabilities:\nNone\n\nRemote-control command(s):\nPOWer:SWITching:RESult:TOTal:ENERgy?"}, {"Level"=4, "Class Only"=FALSE, "Identifier"="RSRTX_ATTR_POWER_SWITCHINGLOSS_MEASUREMENT_TOTAL_POWER_RESULT", "Descriptive Name"="Power Switchingloss Measurement Total Power Result", "Data Type"=1, "Command"="POW:SWIT:RES:TOT:POW?", "Access"=0, "Range Table"="", "Read Callback"="", "Write Callback"="", "Supported Models"="RTM|RTA", "Instrument Options"="", "Flags"=0, "Help"="Result of the measurement\n\nAvailable Repeated Capabilities:\nNone\n\nRemote-control command(s):\nPOWer:SWITching:RESult:TOTal:POWer?"}, {"Level"=2, "Class Only"=TRUE, "Identifier"="", "Descriptive Name"="On Off Measurement", "Data Type"=0, "Command"="", "Access"=0, "Range Table"="", "Read Callback"="", "Write Callback"="", "Supported Models"="", "Instrument Options"="", "Flags"=0, "Help"="Power on/off measurement."}, {"Level"=3, "Class Only"=FALSE, "Identifier"="RSRTX_ATTR_START_POWER_ON_OFF_MEASUREMENT", "Descriptive Name"="Start Power On Off Measurement", "Data Type"=4, "Command"="POW:ONOF:EXEC", "Access"=1, "Range Table"="", "Read Callback"="", "Write Callback"="", "Supported Models"="RTM|RTA", "Instrument Options"="", "Flags"=0, "Help"="Starts the measurement.\n\nAvailable Repeated Capabilities:\nNone\n\nRemote-control command(s):\nPOWer:ONOFf:EXECute"}, {"Level"=3, "Class Only"=FALSE, "Identifier"="RSRTX_ATTR_POWER_ON_OFF_MEASUREMENT_TYPE", "Descriptive Name"="Power On Off Measurement Type", "Data Type"=0, "Command"="POW:ONOF:MEAS", "Access"=2, "Range Table"="rsrtx_rngOnOffType", "Read Callback"="", "Write Callback"="", "Supported Models"="RTM|RTA", "Instrument Options"="", "Flags"=0, "Help"="Configures measurement type.\n\nAvailable Repeated Capabilities:\nNone\n\nRemote-control command(s):\nPOWer:ONOFf:MEASurement"}, {"Level"=3, "Class Only"=FALSE, "Identifier"="RSRTX_ATTR_POWER_ON_OFF_MEASUREMENT_ADD_REPORT", "Descriptive Name"="Power On Off Measurement Add Report", "Data Type"=4, "Command"="POW:ONOF:REP:ADD", "Access"=1, "Range Table"="", "Read Callback"="", "Write Callback"="", "Supported Models"="RTM|RTA", "Instrument Options"="", "Flags"=1, "Help"="Adds the result to the report list.\n\nAvailable Repeated Capabilities:\nNone\n\nRemote-control command(s):\nPOWer:ONOFf:REPort:ADD"}, {"Level"=3, "Class Only"=TRUE, "Identifier"="", "Descriptive Name"="Results", "Data Type"=0, "Command"="", "Access"=0, "Range Table"="", "Read Callback"="", "Write Callback"="", "Supported Models"="", "Instrument Options"="", "Flags"=0, "Help"="Measurement result"}, {"Level"=4, "Class Only"=FALSE, "Identifier"="RSRTX_ATTR_POWER_ON_OFF_MEASUREMENT_RESULT", "Descriptive Name"="Power On Off Measurement Result", "Data Type"=1, "Command"="POW:ONOF:RES{OnOffResult}:TIME?", "Access"=0, "Range Table"="", "Read Callback"="", "Write Callback"="", "Supported Models"="RTM|RTA", "Instrument Options"="", "Flags"=0, "Help"="Result of the measurement\n\nAvailable Repeated Capabilities:\nOnOffResult: OOR1, OOR2, OOR3\r\n\nRemote-control command(s):\nPOWer:ONOFf:RESult<n>:TIME?"}, {"Level"=2, "Class Only"=TRUE, "Identifier"="", "Descriptive Name"="Safe Operating Area", "Data Type"=0, "Command"="", "Access"=0, "Range Table"="", "Read Callback"="", "Write Callback"="", "Supported Models"="", "Instrument Options"="", "Flags"=0, "Help"="Configures the Safe Operating Area.\nThe safe operating area is defined by the voltage and current conditions over which a\npower semiconductor device is expected to operate without self-damage. The &quot;Safe\nOperating Area&quot; analysis provides a diagram of the safe operating conditions of your\ndevice."}, {"Level"=3, "Class Only"=FALSE, "Identifier"="RSRTX_ATTR_START_POWER_SAFE_OPERATING_AREA_MEASUREMENT", 
